vi "Get Terminal Refs for API VI.vi"(8 "error in (no error)":errorcluster, 10 "SubVI ref":refnum<vi>, 11 "Setter Generator In":refnum<class "API VI Generator.lvclass">) -> (0 "error out":errorcluster, 2 "SubVI ref out":refnum<vi>, 3 "Setter Generator Out":refnum<class "API VI Generator.lvclass">)   [LabVIEW 2020, in "Method Generation.lvlib" / "API VI Generator.lvclass"]
uses:
  API VI Generator.lvclass
  API VI Generator.lvclass/API VI Generator.ctl
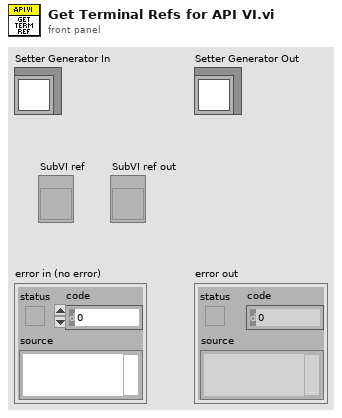
[diagram p1: front panel]
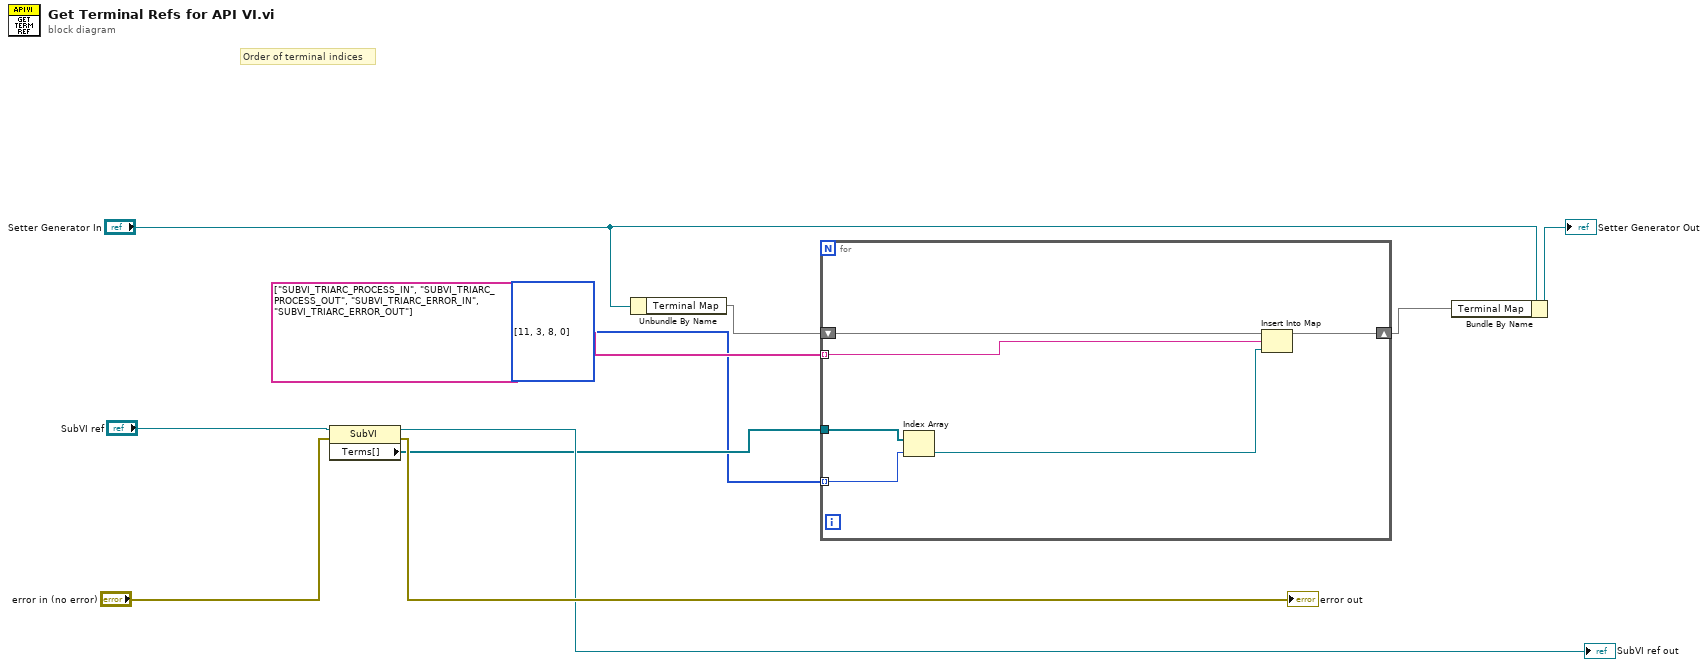
[diagram p0: block diagram]
diagram:
  # "Order of terminal indices"
  n1 = property class="SubVI"(reference="SubVI ref", error in="error in (no error)") -> (reference out=→"SubVI ref out":refnum<vi>, error out=→"error out":errorcluster, "Terms[]"=w2:refnum<vi>[])
  n2 = Unbundle By Name("Setter Generator In") -> ("Terminal Map"=w7:map{string, refnum<vi>})
  n3 = for {
    tunnel: w2 -> [w14]
    tunnel: string[] ["SUBVI_TRIARC_PROCESS_IN", "SUBVI_TRIARC_PROCESS_OUT", "SUBVI_TRIARC_ERROR_IN", "SUBVI_TRIARC_ERROR_OUT"] -> [w16] mode=indexing
    shift-right: [w15] -> w6
    shift-left: w7 -> [w17]
    tunnel: i32[] [11, 3, 8, 0] ("index") -> [w12] mode=indexing
    n4 = Index Array(array=w14, index=w12) -> (element=w13:refnum<vi>)
    n5 = Insert Into Map(map in=w17, key=w16, value=w13) -> (map out=w15:map{string, refnum<vi>})  [unwired: 2 out]
  }
  n6 = Bundle By Name(cluster="Setter Generator In", "Terminal Map"=w6) -> (→"Setter Generator Out":refnum<class "API VI Generator.lvclass">)
